vi "Increment Error Counts.vi"(4 "specific errors":T1, 6 "receiving errors":i16, 7 "channel data offsets":cluster{"error counts":u32}, 11 "values in":dbl[](array[numeric])) -> (3 "values out":dbl[](array[numeric]))   [LabVIEW 2020, in "Ballard ARINC 429 Engine.lvlib" / "Custom Device.lvlib"]
uses:
  Custom Device.lvlib
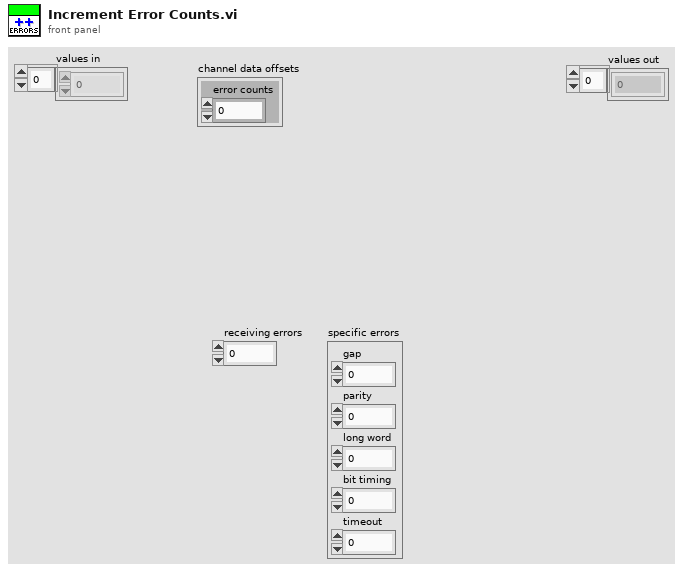
[diagram p1: front panel]
types:
  T1 = cluster{"gap":i16, "parity":i16, "long word":i16, "bit timing":i16, "timeout":i16}
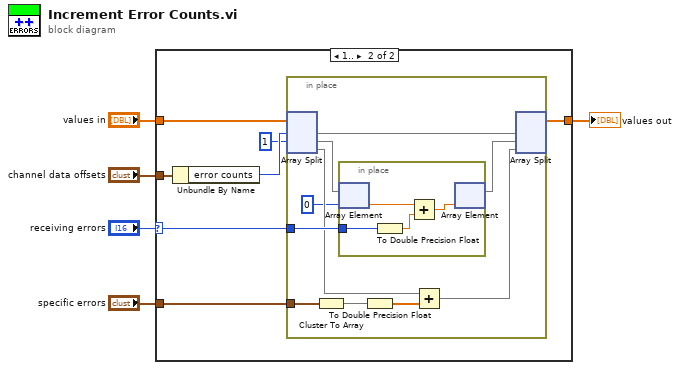
[diagram p0: block diagram]
diagram:
  n1 = case shown="1.." "receiving errors" {
    selector: "receiving errors" -> [_ w12]
    tunnel: "specific errors" -> [_ w13]
    tunnel: "channel data offsets" -> [_ w11]
    tunnel: "values in" -> [w6 w10]
    tunnel: [w6 w8] -> w2
    frame Default {
    }
    frame 1.. {
      n2 = Unbundle By Name(w11) -> ("error counts"=w9:u32)
      n3 = in-place {
        in-place-border: w13 -> [w19]
        in-place-border: w12 -> [w23]
        n4 = in-place-split #1(w10, w9, 1) -> (w22:dbl[], w21:dbl[], w17:dbl[])
        n5 = Cluster To Array(cluster=w19) -> (array=w20:i16[])
        n6 = in-place {
          in-place-border: w23 -> [w27]
          n7 = in-place-array #2(w21, 0) -> (w25:dbl)
          n8 = To Double Precision Float(number=w27) -> (double precision float=w26:dbl)
          n9 = Add(x=w25, y=w26) -> (x+y=w24:dbl)
          n10 = in-place-array #2(w24) -> (w18:dbl[])  [unwired: 1 out]
        }
        n11 = To Double Precision Float(number=w20) -> (double precision float=w16:dbl[])
        n12 = Add(x=w17, y=w16) -> (x+y=w15:dbl[])
        n13 = in-place-split #1(w22, w18, w15) -> (w8:dbl[])  [unwired: 2 out]
      }
    }
  }
  "values out" <- w2
